vi "Toggle Execution Highlighting Probe.vi"() -> (2 "Value String":string, 3 "Boolean":bool)   [LabVIEW 2020]
panel:
  in  "off":string="Execution Highlighting Disabled"
  in  "on":string="Execution Highlighting Enabled"
  out "New Setting":bool
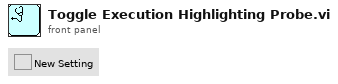
[diagram p1: front panel]
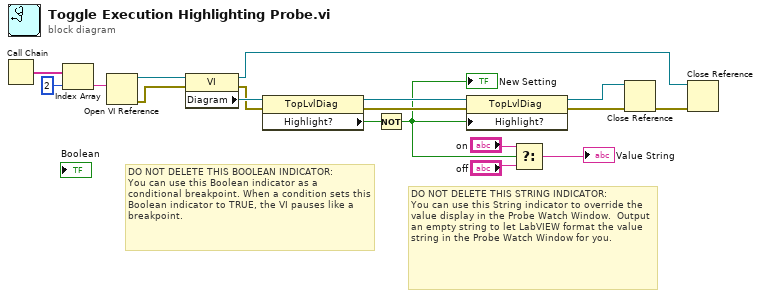
[diagram p0: block diagram]
diagram:
  # "DO NOT DELETE THIS STRING INDICATOR: \nYou can use this String indicator to override the value display in the Probe Watch Window.  Output an empty string to let LabVIEW format the value string in the Probe Watch Window for you."
  # "DO NOT DELETE THIS BOOLEAN INDICATOR: \nYou can use this Boolean indicator as a conditional breakpoint. When a condition sets this Boolean indicator to TRUE, the VI pauses like a breakpoint."
  n1 = Call Chain() -> (call chain=w18:string[])
  n2 = Index Array(array=w18, index=2) -> (element=w16:string)
  n3 = Open VI Reference(vi path=w16) -> (vi reference=w15:refnum<vi>, error out=w12:errorcluster)  [unwired: 5 in]
  n4 = property class="VI"(reference=w15, error in=w12) -> (reference out=w6:refnum<vi>, error out=w13:errorcluster, "Diagram"=w14:refnum<vi>)
  n5 = property class="TopLvlDiag"(reference=w14, error in=w13) -> (reference out=w11:refnum<vi>, error out=w10:errorcluster, "Highlight?"=w5:bool)
  n6 = Not(x=w5) -> (.not. x?=w4:bool)
  "New Setting" <- w4
  n7 = property class="TopLvlDiag"(reference=w11, error in=w10, "Highlight?"=w4) -> (reference out=w8:refnum<vi>, error out=w9:errorcluster)
  n8 = Select(t="on", s=w4, f="off") -> (s? t:f=→"Value String":string)
  n9 = Close Reference(reference=w8, error in (no error)=w9) -> (error out=w7:errorcluster)
  n10 = Close Reference(reference=w6, error in (no error)=w7) -> ()  [unwired: 1 out]
